vi "Curtin1_GetTestListing.vi"(8 "Rebuild":bool, 11 "Type":bool) -> (3 "Array":string[](array[string]))   [LabVIEW 2022 SP3]
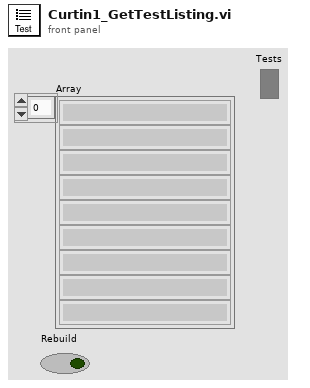
[diagram p1: front panel]
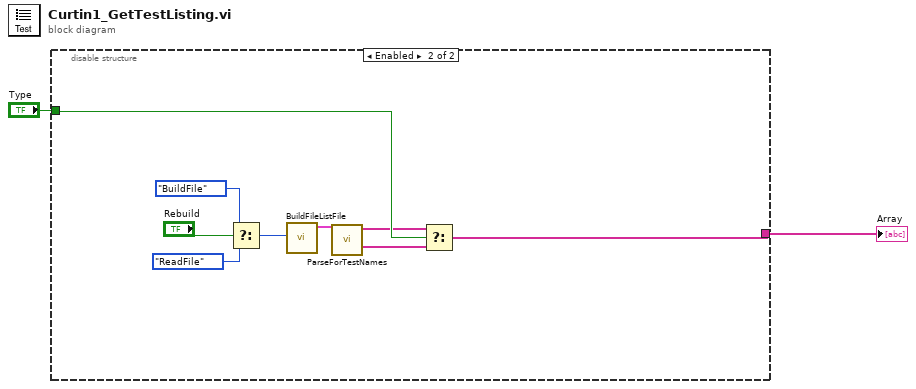
[diagram p0: block diagram]
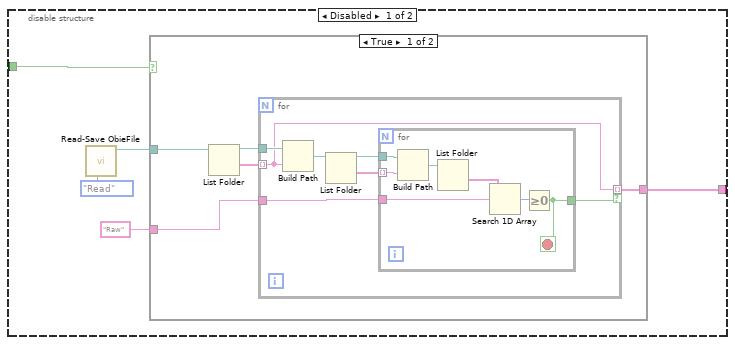
[diagram p2: hidden frame]
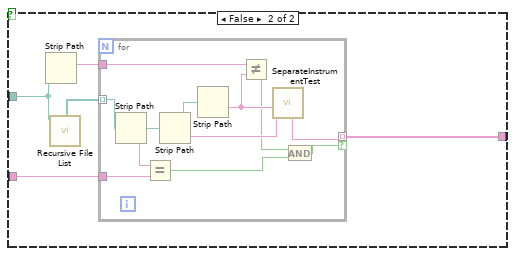
[diagram p3: hidden frame]
diagram:
  n1 = disable-structure shown="Enabled" {
    disable-tunnel: [w7 w48] -> w2
    disable-tunnel: "Type" -> [w4 w51]
    frame Disabled {
      n2 = call "Read-Save ObieFile.vi"("Task"=enum16{"Save", "Read"}."Read") -> ("DataPath Out"=w5:path)  [unwired: 8 in, 2 out]
      n3 = case shown="True" w4 {
        tunnel: [w8 w31] -> w7
        tunnel: w5 -> [w12 w29]
        tunnel: "Raw" ("pattern") -> [w9 w27]
        frame True {
          n4 = List Folder(path=w12) -> (path out=w10:path, folder names=w11:string[])  [unwired: 3 in, 2 out]
          n5 = for {
            tunnel: w11 -> [w15] mode=indexing
            tunnel: w10 -> [w19]
            tunnel: w9 -> [w16]
            tunnel: [w15] -> w8 mode=indexing if=w14
            n6 = Build Path(base path=w19, name or relative path=w15) -> (appended path=w18:path)
            n7 = List Folder(path=w18) -> (path out=w13:path, folder names=w17:string[])  [unwired: 3 in, 2 out]
            n8 = for {
              tunnel: w17 -> [w23] mode=indexing
              tunnel: w16 -> [w26]
              tunnel: [w20] -> w14
              tunnel: w13 -> [w24]
              stop <- w20 stop-if-true
              n9 = Build Path(base path=w24, name or relative path=w23) -> (appended path=w22:path)
              n10 = List Folder(path=w22) -> (folder names=w21:string[])  [unwired: 3 in, 3 out]
              n11 = Search 1D Array(1D array=w21, element=w26) -> (index of element=w25:i32)  [unwired: 1 in]
              n12 = Greater Or Equal To 0?(x=w25) -> (x >= 0?=w20:bool)
            }
          }
        }
        frame False {
          n13 = Strip Path(path=w29) -> (name=w28:string)  [unwired: 1 out]
          n14 = call <vilib>:"Recursive File List.vi"("Folder Path"=w29) -> ("All Folders"=w30:path[])  [unwired: 6 in, 4 out]
          n15 = for {
            tunnel: w30 -> [w43] mode=indexing
            tunnel: [w33] -> w31 mode=indexing if=w34
            tunnel: w28 -> [w38]
            tunnel: w27 -> [w32]
            n16 = Strip Path(path=w43) -> (stripped path=w42:path, name=w41:string)
            n17 = Equal?(x=w41, y=w32) -> (x = y?=w35:bool)
            n18 = Strip Path(path=w42) -> (stripped path=w40:path, name=w39:string)
            n19 = Strip Path(path=w40) -> (name=w37:string)  [unwired: 1 out]
            n20 = Not Equal?(x=w38, y=w37) -> (x != y?=w36:bool)
            n21 = call "SeparateInstrumentTest.vi"("test in"=w39, "Instrument in"=w37) -> ("Instrument -- test out"=w33:string)  [unwired: 5 in, 4 out]
            n22 = And(x=w36, y=w35) -> (x .and. y?=w34:bool)
          }
        }
      }
    }
    frame Enabled {
      n23 = Select(t=enum16{"BuildFile", "ReadFile"}."BuildFile" ("Task"), s="Rebuild", f=enum16{"BuildFile", "ReadFile"}."ReadFile" ("Task")) -> (s? t:f=w44:enum16{"BuildFile", "ReadFile"})
      n24 = call "BuildFileListFile.vi"("Task"=w44) -> ("Instruments"=w52:cluster{"Folder Path":path, "tags":string[]}[])  [unwired: 9 in, 1 out]
      n25 = call "ParseForTestNames.vi"("Instruments"=w52) -> ("tests"=w49:string[], "instruments"=w50:string[])  [unwired: 9 in]
      n26 = Select(t=w50, s=w51, f=w49) -> (s? t:f=w48:string[])
    }
  }
  "Array" <- w2
